vi "Flush Receiver Buffer.vi"(8 "error in (no error)":errorcluster, 11 "EPU452 in":refnum<class "EPU452.lvclass">) -> (0 "error out":errorcluster, 3 "EPU452 out":refnum<class "EPU452.lvclass">)   [LabVIEW 2018, in "EPU452.lvclass"]
uses:
  EPU452.lvclass
  EPU452.lvclass/EPU452.ctl
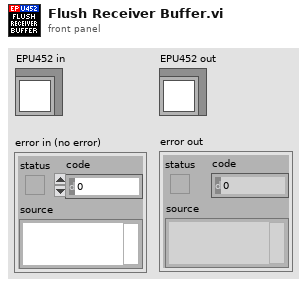
[diagram p1: front panel]
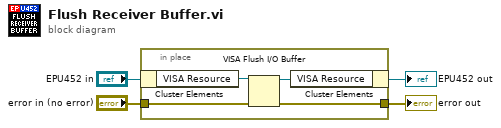
[diagram p0: block diagram]
diagram:
  n1 = in-place {
    in-place-border: "error in (no error)" -> [w6]
    in-place-border: [w5] -> w1
    n2 = in-place-cluster #1("EPU452 in") -> ("VISA Resource"=w8:refnum<visa-resource-name>)
    n3 = VISA Flush I/O Buffer(VISA resource name=w8, error in (no error)=w6) -> (VISA resource name out=w7:refnum<visa-resource-name>, error out=w5:errorcluster)  [unwired: 1 in]
    n4 = in-place-cluster #1("VISA Resource"=w7) -> (→"EPU452 out":refnum<class "EPU452.lvclass">)
  }
  "error out" <- w1
